vi "Print.vi"(8 "error in (no error)":errorcluster caption="entrée d'erreur (pas d'erreur)", 11 "Class Printer_CAB en entrée":refnum<class "Class Printer_TSC.lvclass">) -> (0 "error out":errorcluster caption="sortie d'erreur", 3 "Class Printer_CAB en sortie":refnum<class "Class Printer_TSC.lvclass">)   [LabVIEW 2020, in "Library Instrument & Equipement.lvlib" / "Library Printer.lvlib" / "Class Printer_TSC.lvclass"]
uses:
  Class Printer_TSC.lvclass
  C:/Users/ngarcin/OneDrive - Altyor/Standard TB/Class/Printer/Printer (Default)/Class Printer (Default).lvclass
  Printer (Default)/Class Printer (Default).lvclass
  Class Printer_TSC.lvclass/Class Printer_TSC.ctl
  TSCLIB/TSCLIB.lvlib
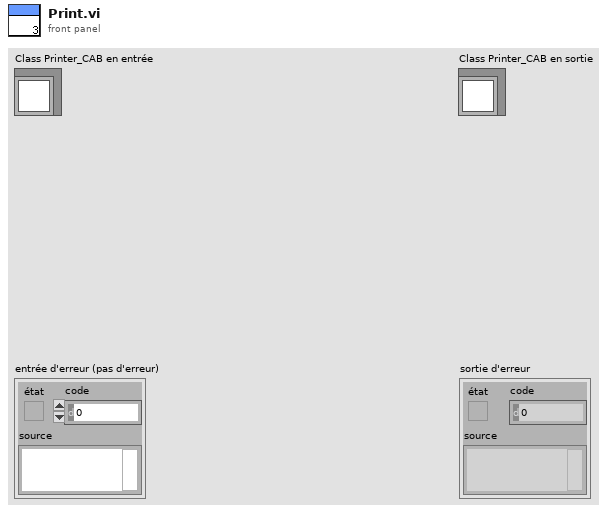
[diagram p1: front panel]
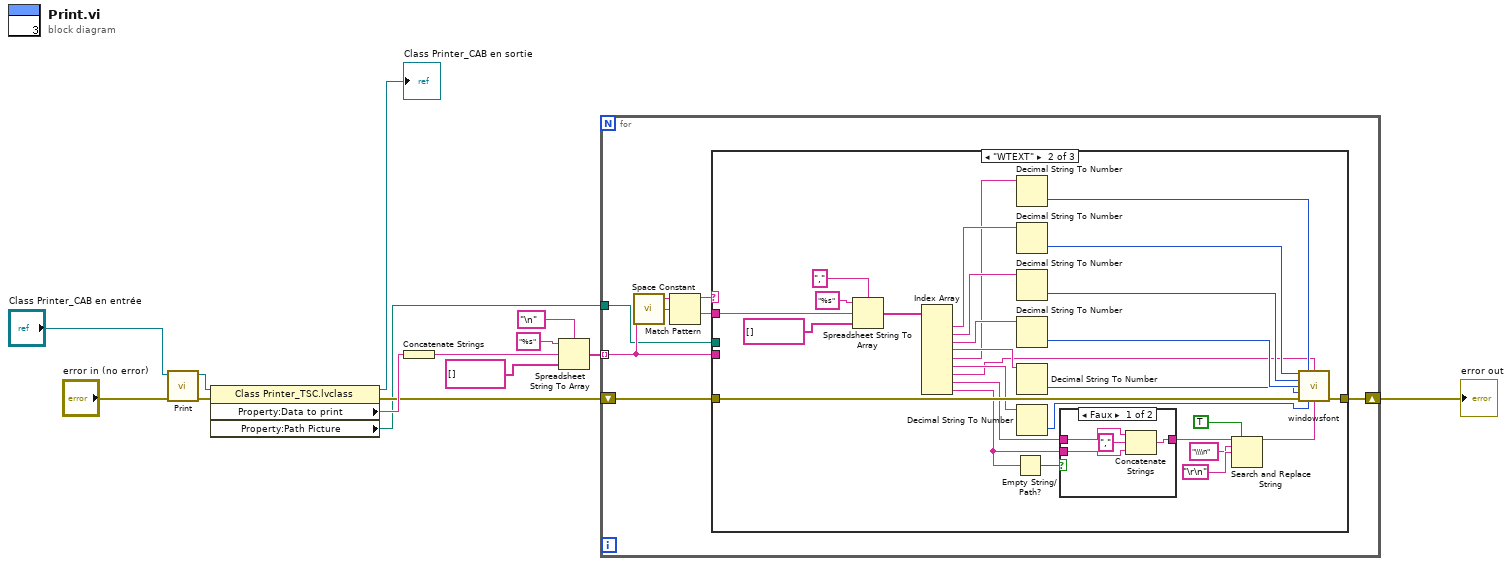
[diagram p0: block diagram]
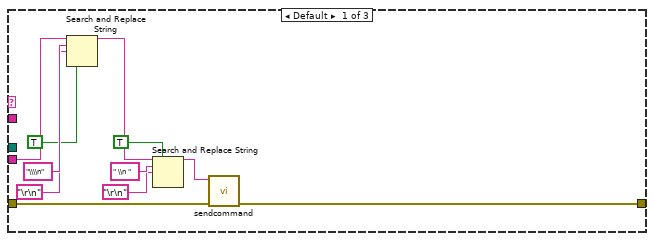
[diagram p2: hidden frame]
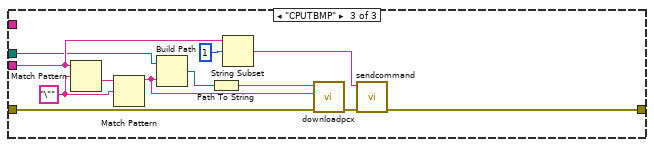
[diagram p4: hidden frame]
diagram:
  n1 = call-parent "Print.vi"("error in (no error)"="error in (no error)", "Class Printer (Default) en entrée"="Class Printer_CAB en entrée") -> ("error out"=w2:errorcluster, "Class Printer (Default) en sortie"=w7:refnum<class "Class Printer_TSC.lvclass">)  [unwired: 8 in]
  n2 = property class="Class Printer_TSC.lvclass"(reference=w7, error in=w2) -> (reference out=→"Class Printer_CAB en sortie":refnum<class "Class Printer_TSC.lvclass">, error out=w4:errorcluster, "Property:Data to print"=w8:string, "Property:Path Picture"=w3:path)
  n3 = Concatenate Strings(w8) -> (w11:string)
  n4 = Spreadsheet String To Array(delimiter (Tab)="\n" ("séparateur (Tabulation)"), format string="%s" ("chaîne de format"), spreadsheet string=w11, array type (2D Dbl)=string[] []) -> (array=w5:string[])
  n5 = for {
    shift-right: [w20] -> w1
    shift-left: w4 -> [w21]
    tunnel: w5 -> [w19] mode=indexing
    tunnel: w3 -> [w15]
    n6 = call <vilib>:"Space Constant.vi"() -> ("String"=w18:string)
    n7 = Match Pattern(string=w19, regular expression=w18) -> (before substring=w17:string, after substring=w16:string)  [unwired: 1 in, 2 out]
    n8 = case shown="\"WTEXT\"" w17 {
      tunnel: w21 -> [w32 w57 w75]
      tunnel: [w31 w56 w77] -> w20
      tunnel: w19 -> [w24 _ w71]
      tunnel: w16 -> [_ w60 _]
      tunnel: w15 -> [_ _ w68]
      frame Default {
        n9 = Search and Replace String(replace all?=TRUE ("tout remplacer ? (F)"), input string=w24, search string="\\\\n" ("chaîne recherchée"), replace string="\r\n") -> (result string=w23:string)  [unwired: 4 in, 3 out]
        n10 = Search and Replace String(replace all?=TRUE ("tout remplacer ? (F)"), input string=w23, search string=" \\n " ("chaîne recherchée"), replace string="\r\n") -> (result string=w30:string)  [unwired: 4 in, 3 out]
        n11 = call "sendcommand.vi"("error in (no error)"=w32, "para0"=w30) -> ("error out"=w31:errorcluster)  [unwired: 7 in, 2 out]
      }
      frame "WTEXT" {
        n12 = Spreadsheet String To Array(delimiter (Tab)="," ("séparateur (Tabulation)"), format string="%s" ("chaîne de format"), spreadsheet string=w60, array type (2D Dbl)=string[] []) -> (array=w55:string[])
        n13 = Index Array(array=w55) -> (element #1=w52:string, element #2=w50:string, element #3=w49:string, element #4=w47:string, element #5=w45:string, element #6=w43:string, element #7=w41:string, element #8=w40:string, element #9=w38:string)  [unwired: 9 in]
        n14 = Empty String/Path?(string/path=w38) -> (empty?=w39:bool)
        n15 = Decimal String To Number(string=w45) -> (number=w44:i32)  [unwired: 2 in, 1 out]
        n16 = Decimal String To Number(string=w52) -> (number=w53:i32)  [unwired: 2 in, 1 out]
        n17 = Decimal String To Number(string=w50) -> (number=w51:i32)  [unwired: 2 in, 1 out]
        n18 = Decimal String To Number(string=w49) -> (number=w48:i32)  [unwired: 2 in, 1 out]
        n19 = Decimal String To Number(string=w47) -> (number=w46:i32)  [unwired: 2 in, 1 out]
        n20 = Decimal String To Number(string=w43) -> (number=w42:i32)  [unwired: 2 in, 1 out]
        n21 = case shown="Faux" w39 {
          tunnel: w38 -> [w64 _]
          tunnel: w40 -> [w63 w65]
          tunnel: [w62 w65] -> w37
          frame False {
            n22 = Concatenate Strings(w63, "," ("chaîne"), w64) -> (w62:string)
          }
          frame True {
          }
        }
        n23 = Search and Replace String(replace all?=TRUE ("tout remplacer ? (F)"), input string=w37, search string="\\\\n" ("chaîne recherchée"), replace string="\r\n") -> (result string=w34:string)  [unwired: 4 in, 3 out]
        n24 = call "windowsfont.vi"("x"=w53, "fontstyle"=w44, "szFaceName"=w41, "y"=w51, "fontheight"=w48, "rotation"=w46, "error in (no error)"=w57, "fontunderline"=w42, "content"=w34) -> ("error out"=w56:errorcluster)  [unwired: 3 in, 3 out]
      }
      frame "CPUTBMP" {
        w72 = "\"" ("chaîne de remplacement (\"\")")
        n25 = Match Pattern(string=w71, regular expression=w72) -> (after substring=w73:string)  [unwired: 1 in, 3 out]
        n26 = Match Pattern(string=w73, regular expression=w72) -> (before substring=w70:string)  [unwired: 1 in, 3 out]
        n27 = Build Path(base path=w68, name or relative path=w70) -> (appended path=w69:path)
        n28 = Path To String(path=w69) -> (string=w66:string)
        n29 = String Subset(string=w71, offset (0)=1) -> (substring=w67:string)  [unwired: 1 in]
        n30 = call "downloadpcx.vi"("error in (no error)"=w75, "image_name"=w70, "filename"=w66) -> ("error out"=w74:errorcluster)  [unwired: 5 in, 3 out]
        n31 = call "sendcommand.vi"("error in (no error)"=w74, "para0"=w67) -> ("error out"=w77:errorcluster)  [unwired: 7 in, 2 out]
      }
    }
  }
  "error out" <- w1
